vi "AMZ_S3_APIHLP_Convert Boolean string to boolean.vi"(4 "Boolean string in":string) -> (1 "Boolean out":bool)   [LabVIEW 2015, in "LV Interface for Amazon S3.lvlib"]
uses:
  LV Interface for Amazon S3.lvlib
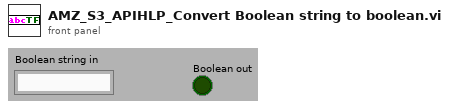
[diagram p1: front panel]
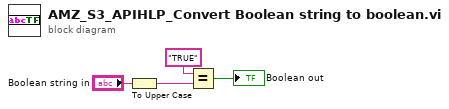
[diagram p0: block diagram]
diagram:
  n1 = To Upper Case(1:"Boolean string in") -> (0:w3:string)
  n2 = Equal?(x="TRUE", y=w3) -> (x = y?=→"Boolean out":bool)
